vi "Flatten Packet Header.vi"(8 "error in (no error)":errorcluster, 9 "Flattened Data in":u8[](array[numeric])=[0, 0, 0, 0, 0, 0, 0, 0] format="%.0x", 10 "Packet Header in":T1, 11 "pcap Parse and Build in":refnum<class "pcap Parse and Build.lvclass">) -> (0 "error out":errorcluster, 1 "Flattened Data out":u8[](array[numeric])=[0, 0, 0, 0, 0, 0, 0, 0, 1, 2, 3, 4, 5], 2 "Packet Header out":T1, 3 "pcap Parse and Build out":refnum<class "pcap Parse and Build.lvclass">)   [LabVIEW 2021, in "pcap Parse and Build.lvclass"]
uses:
  pcap Parse and Build.lvclass
  Typedef/Packet Header.ctl
  e4177ba7-55c0-4140-bea2-15e5e44a53d0.vi
  e4177ba7-55c0-4140-bea2-15e5e44a53d0.vi/c28b0ead-42ad-4072-80a2-aca7f2bd7ce3.vi
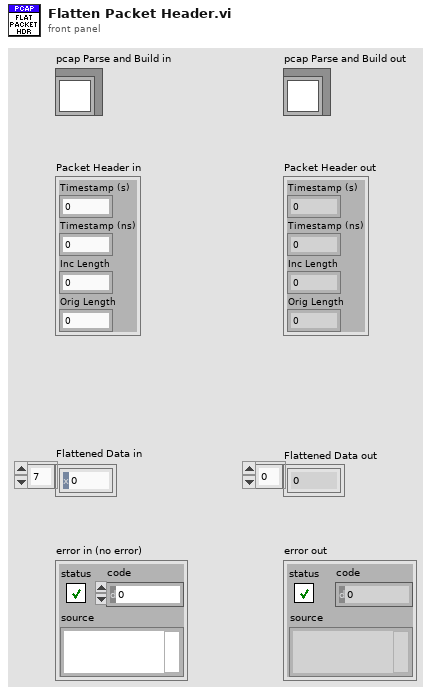
[diagram p1: front panel]
types:
  T1 = typedef "pcap Parse and Build.lvclass/Packet Header.ctl" = cluster{"Timestamp (s)":u32, "Timestamp (ns)":u32, "Inc Length":u32, "Orig Length":u32}
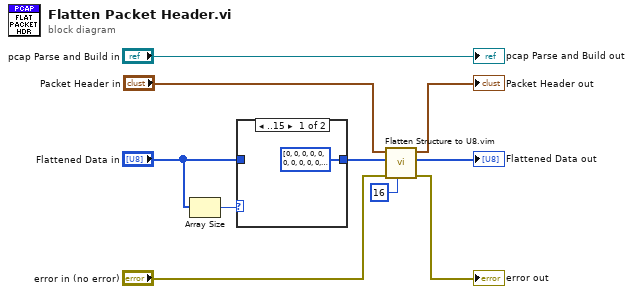
[diagram p0: block diagram]
diagram:
  n1 = Array Size(array="Flattened Data in") -> (size(s)=w6:i32)
  n2 = case shown="..15" w6 {
    tunnel: "Flattened Data in" -> [_ w12]
    tunnel: [u8[] [0, 0, 0, 0, 0, 0, 0, 0, 0, 0, 0, 0, 0, 0, 0, 0] ("Flattened Data in") w12] -> w7
    frame ..15 {
    }
    frame 16, Default {
    }
  }
  n3 = call "Flatten Structure to U8.vim"("Length override"=u64 16, "error in"="error in (no error)", "Flattened Data in"=w7, "Data to Flatten in"="Packet Header in") -> ("error out"=→"error out":errorcluster, "Flattened Data out"=→"Flattened Data out":u8[], "Data to Flatten out"=→"Packet Header out":T1)  [unwired: 5 in]
  "pcap Parse and Build out" <- "pcap Parse and Build in"
